vi "EMCCD external trigger test.vi"() -> ()   [LabVIEW 2018]
panel:
  out "trigger number":i32
  in  "EMCCD trigger port 3":tag="Dev1/port0/line0"
  out "Return from GetStatus 2":u32
  in  "EMCCD trigger port 2":tag="Dev1/port0/line0"
  in  "turn on cooler":bool
  in  "kinetic series":i32=1
  in  "path":string="D:\\YD\\test\\test"
  in  "Temperature":i32=-60
  out "Return from Start Acquisition":u32
  out "Cooling":i32
  out "Return from SetTemperature":u32
  out "Calculated Exposure Value":sgl format="%.2f"
  out "Return from CheckTimings":u32
  in  "Exposure Time (secs)":sgl=0.02 format="%.2f"
  in  "Trigger":u32(ring)=1 items=["Internal", "External"]
  out "Detector Y Pixels":i32
  out "Detector X Pixels":i32
  out "?":i32=1
  out "?":i32=1
  out "Return from Initialize":u32
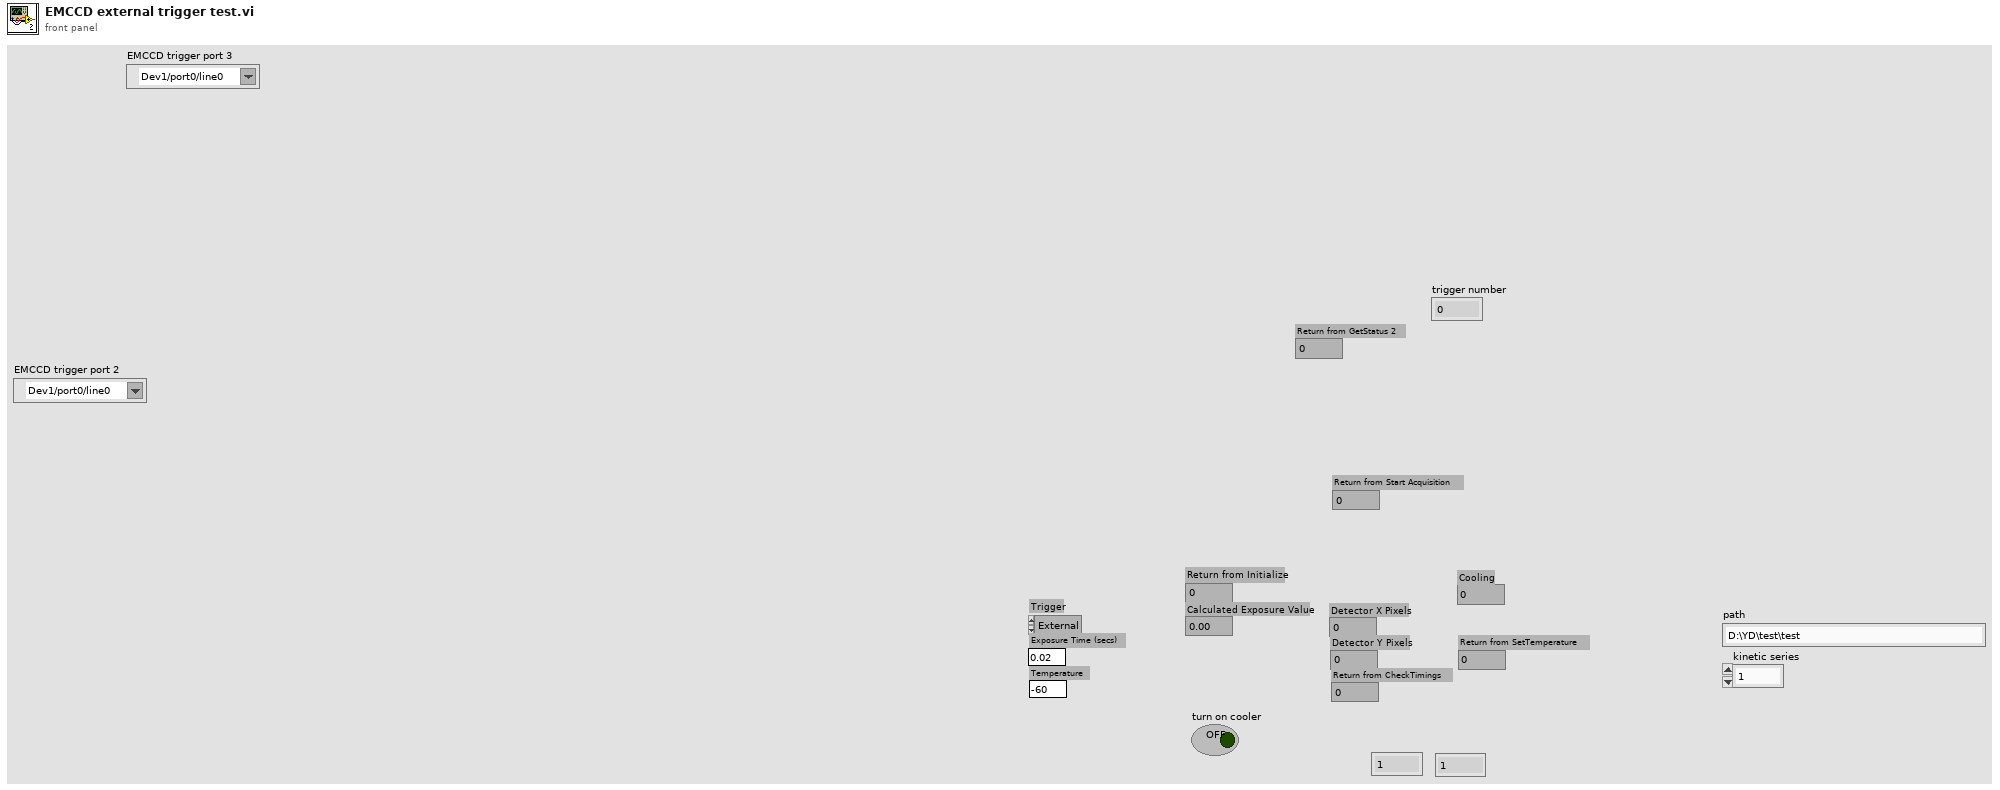
[diagram p1: front panel]
types:
  T1 = typedef "Error Code Enum typedef.ctl" = enum32{"N/A (0)", "DRV_ERROR_CODES", "DRV_SUCCESS", "DRV_VXDNOTINSTALLED", "DRV_ERROR_SCAN", "DRV_ERROR_CHECK_SUM", "DRV_ERROR_FILELOAD", "DRV_UNKNOWN_FUNC", "DRV_ERROR_VXD_INIT", "DRV_ERROR_ADDRESS", "DRV_ERROR_PAGELOCK", "DRV_ERROR_PAGEUNLOCK", "DRV_ERROR_BOARDTEST", "DRV_ERROR_ACK", "DRV_ERROR_UP_FIFO", "DRV_ERROR_PATTERN", "N/A (16)", "DRV_ACQUISITION_ERRORS", "DRV_ACQ_BUFFER", "DRV_ACQ_DOWNFIFO_FULL", "DRV_PROC_UNKONWN_INSTRUCTION", "DRV_ILLEGAL_OP_CODE", "DRV_KINETIC_TIME_NOT_MET", "DRV_ACCUM_TIME_NOT_MET", "DRV_NO_NEW_DATA", "N/A (25)", "DRV_SPOOLERROR", "N/A (27)", "N/A (28)", "N/A (29)", "N/A (30)", "N/A (31)", "N/A (32)", "DRV_TEMPERATURE_CODES", "DRV_TEMPERATURE_OFF", "DRV_TEMPERATURE_NOT_STABILIZED", "DRV_TEMPERATURE_STABILIZED", "DRV_TEMPERATURE_NOT_REACHED", "DRV_TEMPERATURE_OUT_RANGE", "DRV_TEMPERATURE_NOT_SUPPORTED", "DRV_TEMPERATURE_DRIFT", "N/A (41)", "N/A (42)", "N/A (43)", "N/A (44)", "N/A (45)", "N/A (46)", "N/A (47)", "N/A (48)", "DRV_GENERAL_ERRORS", "DRV_INVALID_AUX", "DRV_COF_NOTLOADED", "DRV_FPGAPROG", "DRV_FLEXERROR", "DRV_GPIBERROR", "N/A (55)", "N/A (56)", "N/A (57)", "N/A (58)", "N/A (59)", "N/A (60)", "N/A (61)", "N/A (62)", "N/A (63)", "DRV_DATATYPE", "DRV_DRIVER_ERRORS", "DRV_P1INVALID", "DRV_P2INVALID", "DRV_P3INVALID", "DRV_P4INVALID", "DRV_INIERROR", "DRV_COFERROR", "DRV_ACQUIRING", "DRV_IDLE", "DRV_TEMPCYCLE", "DRV_NOT_INITIALIZED", "DRV_P5INVALID", "DRV_P6INVALID", "DRV_INVALID_MODE", "DRV_INVALID_FILTER", "DRV_I2CERRORS", "DRV_I2CDEVNOTFOUND", "DRV_I2CTIMEOUT", "DRV_P7INVALID", "N/A (84)", "N/A (85)", "N/A (86)", "N/A (87)", "N/A (88)", "N/A (89)", "DRV_IOCERROR", "DRV_VRMVERSIONERROR"}
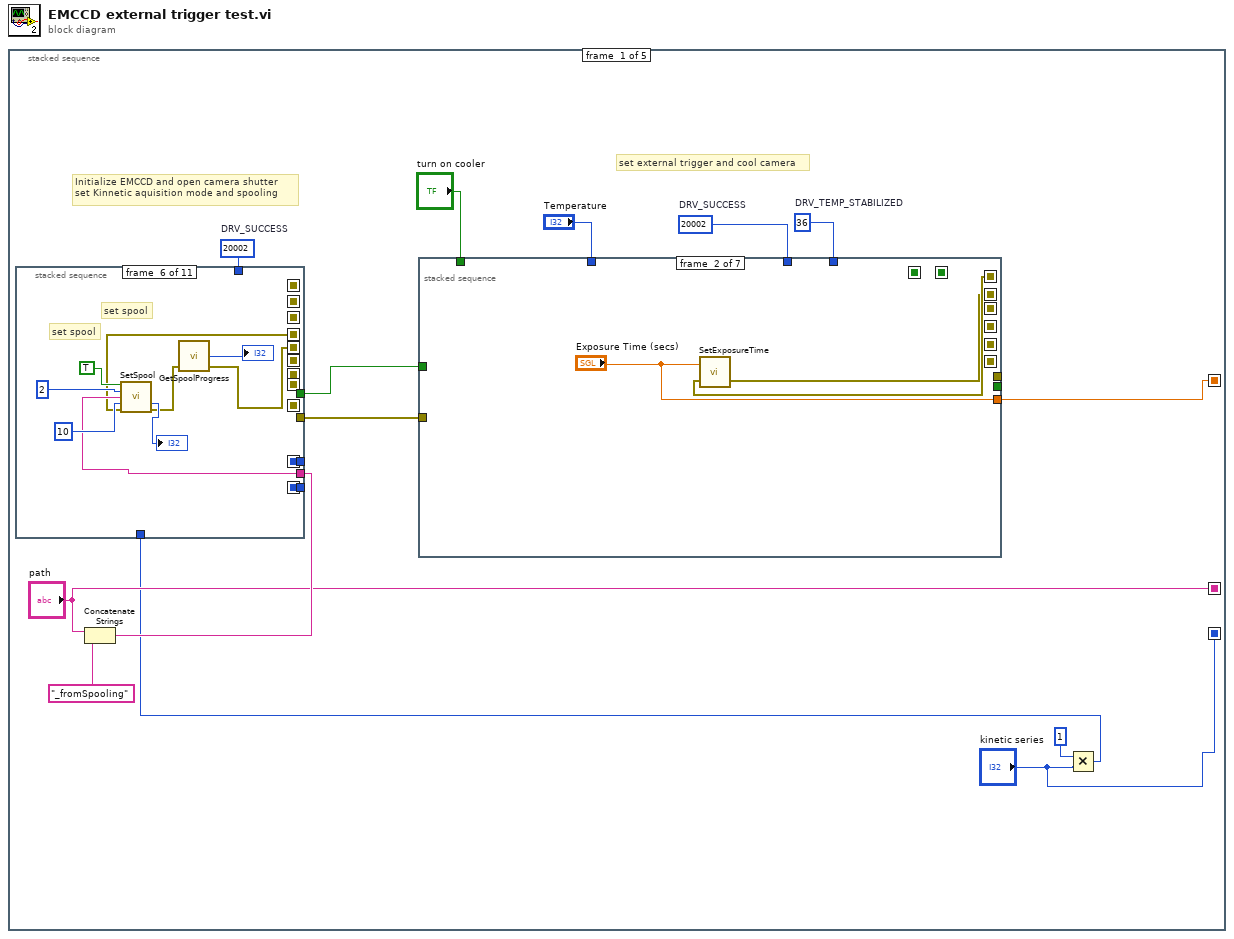
[diagram p0: block diagram]
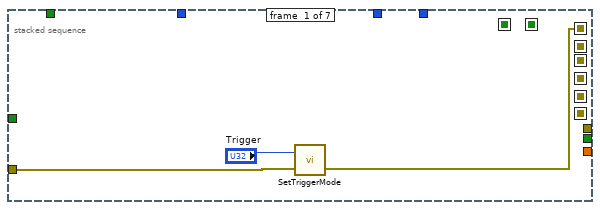
[diagram p2: hidden frame]
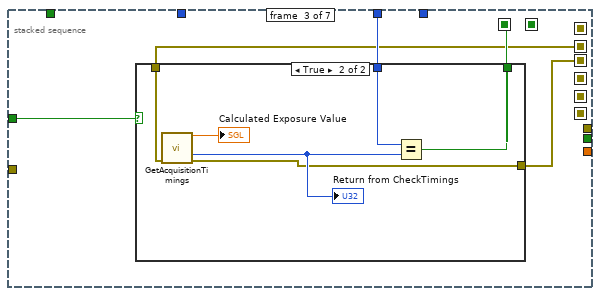
[diagram p3: hidden frame]
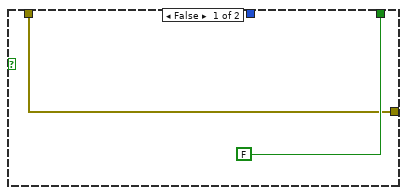
[diagram p4: hidden frame]
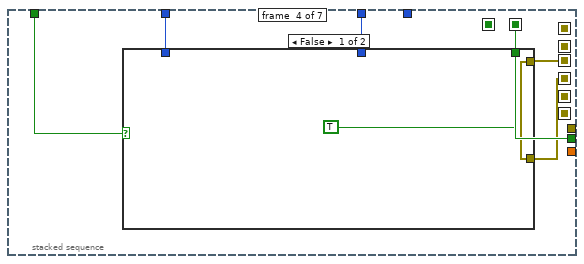
[diagram p5: hidden frame]
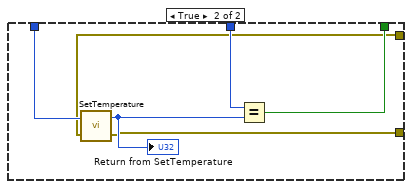
[diagram p6: hidden frame]
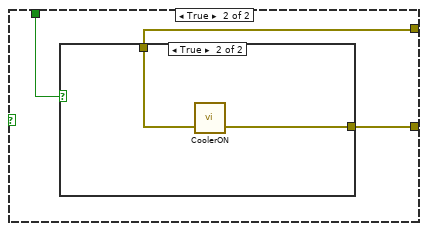
[diagram p8: hidden frame]
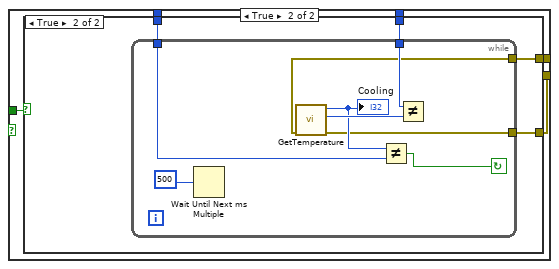
[diagram p11: hidden frame]
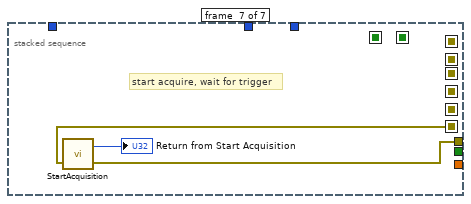
[diagram p13: hidden frame]
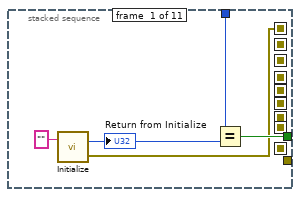
[diagram p14: hidden frame]
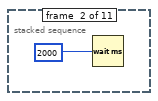
[diagram p15: hidden frame]
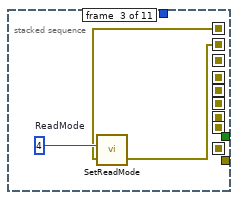
[diagram p16: hidden frame]
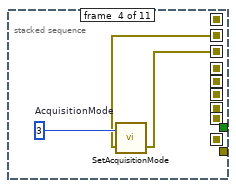
[diagram p17: hidden frame]
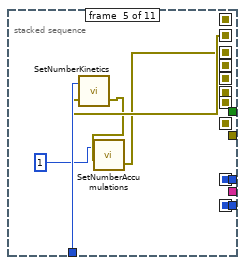
[diagram p18: hidden frame]
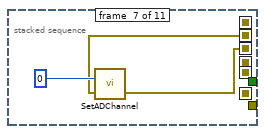
[diagram p19: hidden frame]
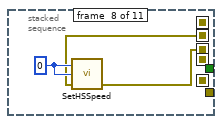
[diagram p20: hidden frame]
diagram:
  n1 = stacked-sequence {
    seq-local: [w8 _ _ _ _] -> [_ w139 _ w158 _]
    seq-local: ["kinetic series" _ _ _ _] -> [_ w137 _ _ _]
    seq-local: ["path" _ _ _ _] -> [_ _ w149 _ _]
    frame #0 {
      w10 = 36  # DRV_TEMP_STABILIZED
      w12 = 20002  # DRV_SUCCESS
      w14 = 20002  # DRV_SUCCESS
      # "set external trigger and cool camera"
      # "Initialize EMCCD and open camera shutter\nset Kinnetic aquisition mode and spooling"
      n2 = Concatenate Strings("path", "_fromSpooling") -> (w5:string)
      n3 = Multiply(x=1, y="kinetic series") -> (x*y=w1:i32)
      n4 = stacked-sequence {
        seq-local: [_ _ _ _ _ _ _ _ _ w130 _] -> [_ _ _ _ _ _ _ _ _ _ _]
        seq-local: [_ _ _ _ _ _ _ _ _ w129 _] -> [_ _ _ _ _ _ _ _ _ _ _]
        seq-local: [w87 _ _ _ _ _ _ _ _ _ _] -> [_ _ w94 _ _ _ _ _ _ _ _]
        seq-local: [_ _ w93 _ _ _ _ _ _ _ _] -> [_ _ _ w97 _ _ _ _ _ _ _]
        seq-local: [_ _ _ w96 _ _ _ _ _ _ _] -> [_ _ _ _ w102 _ _ _ _ _ _]
        seq-local: [_ _ _ _ w100 _ _ _ _ _ _] -> [_ _ _ _ _ w105 _ _ _ _ _]
        seq-local: [_ _ _ _ _ w104 _ _ _ _ _] -> [_ _ _ _ _ _ w114 _ _ _ _]
        seq-local: [_ _ _ _ _ _ w113 _ _ _ _] -> [_ _ _ _ _ _ _ w117 _ _ _]
        seq-local: [_ _ _ _ _ _ _ w116 _ _ _] -> [_ _ _ _ _ _ _ _ w121 _ _]
        seq-local: [_ _ _ _ _ _ _ _ w119 _ _] -> [_ _ _ _ _ _ _ _ _ w128 _]
        seq-local: [_ _ _ _ _ _ _ _ _ w126 _] -> [_ _ _ _ _ _ _ _ _ _ w135]
        tunnel: w14 -> [w89 _ _ _ _ _ _ _ _ _ _]
        tunnel: [w88 _ _ _ _ _ _ _ _ _ _] -> w13
        tunnel: [_ _ _ _ _ _ _ _ _ w130 _] -> _
        tunnel: [_ _ _ _ _ _ _ _ _ w129 _] -> _
        tunnel: w1 -> [_ _ _ _ w103 _ _ _ _ _ _]
        tunnel: w5 -> [_ _ _ _ _ w106 _ _ _ _ _]
        tunnel: [_ _ _ _ _ _ _ _ _ _ w134] -> w9
        frame #0 {
          n5 = call <userlib>:"Initialize.vi"("directory (\"\")"="" ("directory (\"\")")) -> ("error out"=w87:errorcluster, "DLL error code"=w91:u32)  [unwired: 1 in]
          "Return from Initialize" <- w91
          n6 = Equal?(x=w89, y=w91) -> (x = y?=w88:bool)
        }
        frame #1 {
          n7 = Wait (ms)(milliseconds to wait=u32 2000) -> ()  [unwired: 1 out]
        }
        frame #2 {
          w95 = u16 4  # ReadMode
          n8 = call <userlib>:"SetReadMode.vi"("error in (no error)"=w94, "mode"=w95) -> ("error out"=w93:errorcluster)  [unwired: 1 out]
        }
        frame #3 {
          w98 = u16 3  # AcquisitionMode
          n9 = call <userlib>:"SetAcquisitionMode.vi"("error in (no error)"=w97, "mode"=w98) -> ("error out"=w96:errorcluster)  [unwired: 1 out]
        }
        frame #4 {
          n10 = call <userlib>:"SetNumberKinetics.vi"("error in (no error)"=w102, "number"=w103) -> ("error out"=w101:errorcluster)  [unwired: 1 out]
          n11 = call <userlib>:"SetNumberAccumulations.vi"("error in (no error)"=w101, "number"=1) -> ("error out"=w100:errorcluster)  [unwired: 1 out]
        }
        frame #5 {
          # "set spool"
          # "set spool"
          n12 = call <userlib>:"SetSpool.vi"("active"=TRUE, "method"=2, "name"=w106, "framebuffersize (10)"=10, "error in (no error)"=w105) -> ("DLL error code"=→"?":u32, "error out"=w108:errorcluster)  [unwired: 9 in]
          n13 = call <userlib>:"GetSpoolProgress.vi"("error in (no error)"=w108) -> ("error out"=w104:errorcluster, "index"=→"?":i32)  [unwired: 2 in, 1 out]
        }
        frame #6 {
          n14 = call <userlib>:"SetADChannel.vi"("error in (no error)"=w114, "channel"=0) -> ("error out"=w113:errorcluster)  [unwired: 1 out]
        }
        frame #7 {
          w118 = 0
          n15 = call <userlib>:"SetHSSpeed.vi"("error in (no error)"=w117, "index"=w118, "type"=w118) -> ("error out"=w116:errorcluster)  [unwired: 1 in, 1 out]
        }
        frame #8 {
          n16 = call <userlib>:"GetNumberVSSpeeds.vi"("error in (no error)"=w121) -> ("error out"=w120:errorcluster, "number"=w124:i32)  [unwired: 2 in, 1 out]
          n17 = Subtract(x=w124, y=1) -> (x-y=w122:i32)
          n18 = call <userlib>:"SetVSSpeed.vi"("error in (no error)"=w120, "index"=w122) -> ("error out"=w119:errorcluster)  [unwired: 1 out]
        }
        frame #9 {
          w125 = 1002
          w131 = 1
          n19 = call <userlib>:"GetDetector.vi"("error in (no error)"=w128) -> ("error out"=w127:errorcluster, "ypixels"=w130:i32, "xpixels"=w129:i32)  [unwired: 3 in, 1 out]
          "Detector Y Pixels" <- w130
          "Detector X Pixels" <- w129
          n20 = call <userlib>:"SetImage.vi"("hbin"=w131, "vbin"=w131, "hstart"=w131, "hend"=w125, "vstart"=w131, "vend"=w125, "error in (no error)"=w127) -> ("error out"=w126:errorcluster)  [unwired: 19 in, 1 out]
        }
        frame #10 {
          w133 = 0
          w132 = 1
          n21 = call <userlib>:"SetShutter.vi"("type"=w132, "mode"=w132, "closingtime"=w133, "openingtime"=w133, "error in (no error)"=w135) -> ("error out"=w134:errorcluster)  [unwired: 9 in, 1 out]
        }
      }
      n22 = stacked-sequence {
        seq-local: [_ _ w23 _ _ _ _] -> [_ _ _ _ _ _ _]
        seq-local: [_ _ _ w37 _ _ _] -> [_ _ _ _ w51 w63 _]
        seq-local: [w15 _ _ _ _ _ _] -> [_ w20 _ _ _ _ _]
        seq-local: [_ w19 _ _ _ _ _] -> [_ _ w22 _ _ _ _]
        seq-local: [_ _ w21 _ _ _ _] -> [_ _ _ w36 _ _ _]
        seq-local: [_ _ _ w35 _ _ _] -> [_ _ _ _ w50 _ _]
        seq-local: [_ _ _ _ w49 _ _] -> [_ _ _ _ _ w61 _]
        seq-local: [_ _ _ _ _ w60 _] -> [_ _ _ _ _ _ w85]
        tunnel: w12 -> [_ _ w25 w39 _ _ _]
        tunnel: "Temperature" -> [_ _ _ w38 _ w62 _]
        tunnel: w10 -> [_ _ _ _ _ w64 _]
        tunnel: [_ _ _ w37 _ _ _] -> _
        tunnel: w13 -> [_ _ w24 _ _ _ _]
        tunnel: w9 -> [w16 _ _ _ _ _ _]
        tunnel: [_ _ _ _ _ _ w84] -> _
        tunnel: [_ "Exposure Time (secs)" _ _ _ _ _] -> w8
        tunnel: "turn on cooler" -> [_ _ _ w34 w48 w59 _]
        frame #0 {
          n23 = call <userlib>:"SetTriggerMode.vi"("error in (no error)"=w16, "mode"="Trigger") -> ("error out"=w15:errorcluster)  [unwired: 1 out]
        }
        frame #1 {
          n24 = call <userlib>:"SetExposureTime.vi"("error in (no error)"=w20, "time"="Exposure Time (secs)") -> ("error out"=w19:errorcluster)  [unwired: 1 out]
        }
        frame #2 {
          n25 = case shown="True" w24 {
            tunnel: w25 -> [_ w31]
            tunnel: [FALSE w33] -> w23
            tunnel: w22 -> [w26 w29]
            tunnel: [w26 w28] -> w21
            frame False {
            }
            frame True {
              n26 = call <userlib>:"GetAcquisitionTimings.vi"("error in (no error)"=w29) -> ("exposure"=→"Calculated Exposure Value":sgl, "DLL error code"=w30:u32, "error out"=w28:errorcluster)  [unwired: 10 in, 2 out]
              "Return from CheckTimings" <- w30
              n27 = Equal?(x=w31, y=w30) -> (x = y?=w33:bool)
            }
          }
        }
        frame #3 {
          n28 = case shown="False" w34 {
            tunnel: w39 -> [_ w47]
            tunnel: w38 -> [_ w45]
            tunnel: [TRUE w44] -> w37
            tunnel: w36 -> [w40 w43]
            tunnel: [w40 w42] -> w35
            frame False {
            }
            frame True {
              n29 = call <userlib>:"SetTemperature.vi"("error in (no error)"=w43, "temperature"=w45) -> ("error out"=w42:errorcluster, "DLL error code"=w46:u32)
              "Return from SetTemperature" <- w46
              n30 = Equal?(x=w47, y=w46) -> (x = y?=w44:bool)
            }
          }
        }
        frame #4 {
          n31 = case shown="False" w48 {
            tunnel: w51 -> [_ w55]
            tunnel: w50 -> [w52 w54]
            tunnel: [w52 w53] -> w49
            frame False {
            }
            frame True {
              n32 = case shown="True" w55 {
                tunnel: w54 -> [w56 w58]
                tunnel: [w56 w57] -> w53
                frame False {
                }
                frame True {
                  n33 = call <userlib>:"CoolerON.vi"("error in (no error)"=w58) -> ("error out"=w57:errorcluster)  [unwired: 1 in, 1 out]
                }
              }
            }
          }
        }
        frame #5 {
          n34 = case shown="False" w59 {
            tunnel: w64 -> [_ w70]
            tunnel: w63 -> [_ w69]
            tunnel: w62 -> [_ w68]
            tunnel: w61 -> [w65 w67]
            tunnel: [w65 w66] -> w60
            frame False {
            }
            frame True {
              n35 = case shown="True" w69 {
                tunnel: w70 -> [_ w75]
                tunnel: w68 -> [_ w74]
                tunnel: w67 -> [w71 w73]
                tunnel: [w71 w72] -> w66
                frame False {
                }
                frame True {
                  n36 = while {
                    tunnel: w75 -> [w82]
                    tunnel: w74 -> [w79]
                    tunnel: w73 -> [w77]
                    tunnel: [w76] -> w72
                    stop <- w78 continue-if-true
                    n37 = Wait Until Next ms Multiple(millisecond multiple=u32 500) -> ()  [unwired: 1 out]
                    n38 = call <userlib>:"GetTemperature.vi"("error in (no error)"=w77) -> ("error out"=w76:errorcluster, "status"=w81:T1, "temperature"=w80:i32)  [unwired: 3 in, 1 out]
                    "Cooling" <- w80
                    n39 = Not Equal?(x=w80, y=w79) -> (x != y?=w78:bool)
                    n40 = Not Equal?(x=w82, y=w81) -> ()  [unwired: 1 out]
                  }
                }
              }
            }
          }
        }
        frame #6 {
          # "start acquire, wait for trigger"
          n41 = call <userlib>:"StartAcquisition.vi"("error in (no error)"=w85) -> ("error out"=w84:errorcluster, "DLL error code"=→"Return from Start Acquisition":u32)  [unwired: 1 in]
        }
      }
    }
    frame #1 {
      n42 = Add(x=w137, y=2) -> (x+y=w138:i32)
      n43 = for {
        N: w138 -> [_]
        tunnel: w139 -> [w141]
        i -> [w140]
        n44 = stacked-sequence {
          tunnel: w141 -> [w142]
          frame #0 {
            n45 = Add(x=w142, y=0.04) -> (x+y=w144:dbl)
            n46 = Multiply(x=w144, y=1000.0) -> (x*y=w143:dbl)
            n47 = call "trig EMCCD.vi"("exp time (ms)"=w143, "lines"="EMCCD trigger port 2") -> ()  [unwired: 1 in, 1 out]
          }
        }
        "trigger number" <- w140
      }
    }
    frame #2 {
      n48 = case shown="True" TRUE {
        tunnel: w149 -> [w150 w155]
        frame False {
          n49 = call <userlib>:"SaveAsSif.vi"("path"=w150) -> ()  [unwired: 1 in, 2 out]
        }
        frame True {
          n50 = Concatenate Strings(w155, "_fromSaveAsTiff.tif") -> (w153:string)
          n51 = call <userlib>:"SaveAsTiff.vi"("path"=w153, "palette"="C:\\Program Files\\Andor SOLIS\\GREY.PAL", "position"=0, "type"=1) -> ()  [unwired: 10 in, 2 out]
        }
      }
    }
    frame #3 {
      n52 = case shown="True" FALSE {
        tunnel: w158 -> [_ w159]
        frame False {
        }
        frame True {
          n53 = while {
            tunnel: w159 -> [w160]
            stop <- w161 continue-if-true
            n54 = stacked-sequence {
              tunnel: [w163 _] -> w161
              tunnel: w160 -> [_ w165]
              frame #0 {
                w164 = u16 72  # DRV ACQUIRING
                n55 = call <userlib>:"GetStatus.vi"() -> ("status"=w162:T1)  [unwired: 3 in, 2 out]
                "Return from GetStatus 2" <- w162
                n56 = Equal?(x=w162, y=w164) -> (x = y?=w163:bool)
              }
              frame #1 {
                n57 = Add(x=w165, y=0.04) -> (x+y=w167:dbl)
                n58 = Multiply(x=w167, y=1000.0) -> (x*y=w166:dbl)
                n59 = call "trig EMCCD.vi"("exp time (ms)"=w166, "lines"="EMCCD trigger port 3") -> ()  [unwired: 1 in, 1 out]
              }
            }
          }
        }
      }
    }
    frame #4 {
      # "shut down EMCCD"
      n60 = call <userlib>:"ShutDown.vi"() -> ()  [unwired: 2 in, 2 out]
    }
  }
